vi "CRYPEAQ Init.vi"(11 "Fs":dbl=44100.0) -> (2 "Block Size":i32, 3 "Hanning Window":dbl[](array[numeric]))   [LabVIEW 2013]
uses:
  CRYPEAQ Global.vi
panel:
  in  "PCinit":dbl
  in  "Correlation Point Number":dbl=2048.0
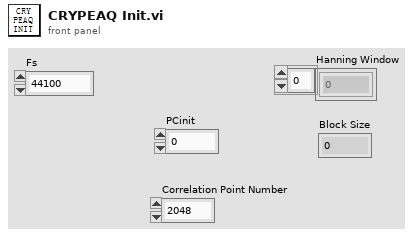
[diagram p1: front panel]
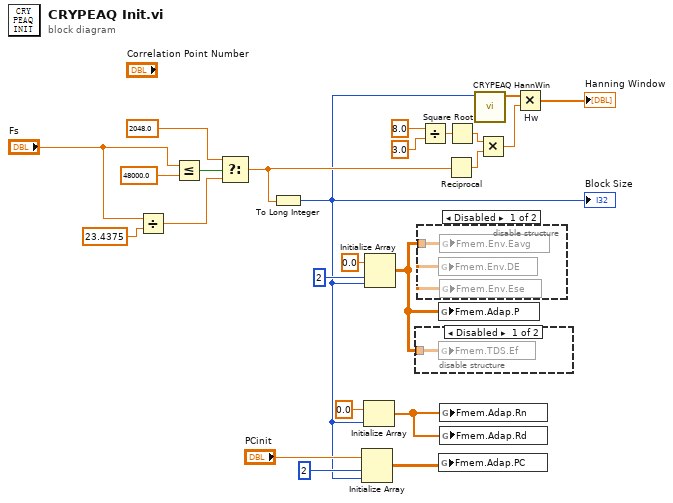
[diagram p0: block diagram]
diagram:
  n1 = Divide(x="Fs", y=23.4375) -> (x/y=w3:dbl)
  n2 = Less Or Equal?(x="Fs", y=48000.0 ("Fs")) -> (x <= y?=w7:bool)
  n3 = Select(t=2048.0 ("Fs"), s=w7, f=w3) -> (s? t:f=w2:dbl)
  n4 = To Long Integer(number=w2) -> (32bit integer=w1:i32)
  "Block Size" <- w1
  n5 = Initialize Array("PCinit", 2 ("dimension size"), w1) -> (w16:dbl[][])
  n6 = Initialize Array(0.0 ("element"), w1) -> (w15:dbl[])
  n7 = Initialize Array(0.0 ("element"), 2 ("dimension size"), w1) -> (w17:dbl[][])
  n8 = disable-structure shown="Disabled" {
    disable-tunnel: w17 -> [w25 _]
    frame Disabled {
      n9 = global write "CRYPEAQ Global.vi" "Fmem.TDS.Ef"(w25) -> ()
    }
    frame Enabled {
    }
  }
  n10 = disable-structure shown="Disabled" {
    disable-tunnel: w17 -> [w26 _]
    frame Disabled {
      n11 = global write "CRYPEAQ Global.vi" "Fmem.Env.DE"(w26) -> ()
      n12 = global write "CRYPEAQ Global.vi" "Fmem.Env.Eavg"(w26) -> ()
      n13 = global write "CRYPEAQ Global.vi" "Fmem.Env.Ese"(w26) -> ()
    }
    frame Enabled {
    }
  }
  n14 = Divide(x=8.0, y=3.0) -> (x/y=w10:dbl)
  n15 = global write "CRYPEAQ Global.vi" "Fmem.Adap.P"(w17) -> ()
  n16 = global write "CRYPEAQ Global.vi" "Fmem.Adap.PC"(w16) -> ()
  n17 = global write "CRYPEAQ Global.vi" "Fmem.Adap.Rn"(w15) -> ()
  n18 = global write "CRYPEAQ Global.vi" "Fmem.Adap.Rd"(w15) -> ()
  n19 = Reciprocal(x=w2) -> (1/x=w12:dbl)
  n20 = Square Root(x=w10) -> (sqrt(x)=w11:dbl)
  n21 = call "CRYPEAQ HannWin.vi"("NF"=w1) -> ("hw"=w14:dbl[])  [unwired: 10 in]
  n22 = Multiply(x=w11, y=w12) -> (x*y=w13:dbl)
  n23 = Multiply "Hw"(x=w14, y=w13) -> (x*y=→"Hanning Window":dbl[])
